vi "log analysis_gps.vi"() -> ()   [LabVIEW 2019] (continued)
02000000,471d,15824;INS_ALIGNMENT_COMPLETE,INS_RTKFIXED,37.37068318728,126.72136703307,8.7806,22.3000,0.4101,0.2924,-0.0105,-0.304454074,-0.851881109,32.302829580,0.4173,0.2841,0.5455,0.1136,0.0938,0.0834,0.2704,0.2490,5.0951,0f000001,0*5034c2f1\n\tsystem status\tnormal 2 28.200000 0 0\trobot status\t47.117309\t61.373325\t8.780600\t-0.304454\t-0.851881\t55.895889\t0.504000\t-0.016000\n\t\n15:08:15.2\tlog_raw\tgps_raw\t\tsystem status\tnormal 2 28.200000 0 0\trobot status\t47.257142\t61.573715\t8.772200\t-0.417275\t-0.794450\t55.326847\t0.500000\t-0.019000\n\t\n15:08:15.7\tlog_raw\tgps_raw\t\tsystem status\tnormal 2 28.200000 0 0\trobot status\t47.399461\t61.774255\t8.766600\t-0.526161\t-1.084867\t54.437000\t0.504000\t-0.024000\n\t\n15:08:16.2\tlog_raw\tgps_raw\t#INSPVAXA,USB3,0,45.5,FINESTEERING,2107,281314.250,02000000,471d,15824;INS_ALIGNMENT_COMPLETE,INS_RTKFIXED,37.37068860278,126.72137185474,8.7599,22.3000,0.3783,0.2883,-0.0099,-0.473451897,-1.199118445,33.419872159,0.4114,0.2852,0.5433,0.1126,0.0924,0.0813,0.2701,0.2485,5.0982,0f000001,0*254465a8\n\tsystem status\tnormal 2 28.200000 0 0\trobot status\t47.544405\t61.974360\t8.759900\t-0.473452\t-1.199118\t53.699936\t0.553000\t0.088000\n\t\n15:08:16.7\tlog_raw\tgps_raw\t#INSPVAXA,USB3,0,45.5,FINESTEERING,2107,281314.750,02000000,471d,15824;INS_ALIGNMENT_COMPLETE,INS_RTKFIXED,37.37069038063,126.72137348955,8.7529,22.3000,0.4019,0.3010,-0.0013,-0.576554942,-1.350073245,33.962253064,0.4114,0.2852,0.5433,0.1126,0.0924,0.0813,0.2701,0.2485,5.0982,0f000001,0*70de1d9e\n\tsystem status\tnormal 2 28.200000 0 0\trobot status\t47.689214\t62.171673\t8.752900\t-0.576555\t-1.350073\t53.539288\t0.494000\t-0.014000\n\t\n15:08:17.2\tlog_raw\tgps_raw\t\tsystem status\tnormal 2 28.200000 0 0\trobot status\t47.833567\t62.364346\t8.744900\t-0.295645\t-1.375257\t53.025951\t0.518000\t-0.006000\n\t\n15:08:17.7\tlog_raw\tgps_raw\t\tsystem status\tnormal 2 28.200000 0 0\trobot status\t47.974700\t62.554374\t8.738100\t-0.566007\t-1.595691\t51.924320\t0.511000\t0.009000\n\t\n15:08:18.2\tlog_raw\tgps_raw\t#INSPVAXA,USB3,0,50.0,FINESTEERING,2107,281316.250,02000000,471d,15824;INS_ALIGNMENT_COMPLETE,INS_RTKFIXED,37.37069553748,126.72137835296,8.7291,22.3000,0.3690,0.3016,-0.0165,-0.475362397,-1.709507066,35.267633649,0.4099,0.2844,0.5412,0.1123,0.0915,0.0796,0.2698,0.2480,5.0999,0f000001,0*7a9fb179\n\tsystem status\tnormal 2 28.200000 0 0\trobot status\t48.120006\t62.744002\t8.729100\t-0.475362\t-1.709507\t52.502842\t0.422000\t-0.071000\n\t\n15:08:18.7\tlog_raw\tgps_raw\t\tsystem status\tnormal 2 28.200000 0 0\trobot status\t48.271629\t62.938231\t8.721200\t-0.350668\t-1.662772\t52.101021\t0.431000\t-0.101000\n\t\n15:08:19.2\tlog_raw\tgps_raw\t#INSPVAXA,USB3,0,50.5,FINESTEERING,2107,281317.250,02000000,471d,15824;INS_ALIGNMENT_COMPLETE,INS_RTKFIXED,37.37069888473,126.72138166049,8.7140,22.3000,0.4002,0.3322,-0.0336,-0.163313359,-1.347458535,36.032748786,0.4094,0.2836,0.5396,0.1129,0.0921,0.0802,0.2696,0.2478,5.0996,0f000001,0*7e476d51\n\tsystem status\tnormal 2 28.200000 0 0\trobot status\t48.412982\t63.115493\t8.714000\t-0.163313\t-1.347459\t51.751701\t0.514000\t-0.007000\n\t\n15:08:19.7\tlog_raw\tgps_raw\t\tsystem status\tnormal 2 28.200000 0 0\trobot status\t48.561151\t63.300949\t8.706600\t-0.217369\t-1.146601\t51.645607\t0.473000\t-0.029000\n\t\n15:08:20.2\tlog_raw\tgps_raw\t#INSPVAXA,USB3,0,50.0,FINESTEERING,2107,281318.250,02000000,471d,15824;INS_ALIGNMENT_COMPLETE,INS_RTKFIXED,37.37070219067,126.72138499710,8.7014,22.3000,0.3959,0.3213,-0.0090,-0.394966992,-1.322496913,36.727773169,0.4088,0.2828,0.5369,0.1123,0.0917,0.0794,0.2695,0.2477,5.0989,0f000001,0*0ac65207\n\tsystem status\tnormal 2 28.200000 0 0\trobot status\t48.708533\t63.482400\t8.701400\t-0.394967\t-1.322497\t51.157326\t0.491000\t-0.005000\n\t\n15:08:20.7\tlog_raw\tgps_raw\t\tsystem status\tnormal 2 28.300000 0 0\trobot status\t48.862404\t63.669120\t8.695100\t-0.380069\t-1.561037\t50.880112\t0.497000\t0.006000\n\t\n15:08:21.2\tlog_raw\tgps_raw\t\tsystem status\tnormal 2 28.200000 0 0\trobot status\t49.009867\t63.846230\t8.690900\t-0.406987\t-1.733069\t50.231125\t0.491000\t0.004000\n\t\n15:08:21.7\tlog_raw\tgps_raw\t#INSPVAXA,USB3,0,48.5,FINESTEERING,2107,281319.750,02000000,471d,15824;INS_ALIGNMENT_COMPLETE,INS_RTKFIXED,37.37070705981,126.72139005862,8.6887,22.3000,0.3656,0.3184,-0.0246,-0.462020881,-1.503034844,37.411185291,0.4083,0.2820,0.5343,0.1120,0.0915,0.0787,0.2694,0.2475,5.0983,0f000001,0*abb76b38\n\tsystem status\tnormal 2 28.300000 0 0\trobot status\t49.156875\t64.022797\t8.688700\t-0.462021\t-1.503035\t50.616264\t0.494000\t0.013000\n\t\n15:08:22.2\tlog_raw\tgps_raw\t\tsystem status\tnormal 2 28.200000 0 0\trobot status\t49.308245\t64.205716\t8.683800\t-0.851405\t-1.203471\t49.388012\t0.496000\t0.022000\n\t\n15:08:22.7\tlog_raw\tgps_raw\t#INSPVAXA,USB3,0,48.5,FINESTEERING,2107,281320.750,02000000,471d,15824;INS_ALIGNMENT_COMPLETE,INS_RTKFIXED,37.37071031528,126.72139346401,8.6801,22.3000,0.3719,0.3343,-0.0256,-0.836621928,-1.161971448,37.866051675,0.4083,0.2824,0.5333,0.1117,0.0916,0.0783,0.2693,0.2474,5.0979,0f000001,0*4c0e47a3\n\tsystem status\tnormal 2 28.200000 0 0\trobot status\t49.458518\t64.384102\t8.680100\t-0.836622\t-1.161971\t50.094471\t0.500000\t-0.004000\n\t\n15:08:23.2\tlog_raw\tgps_raw\t\tsystem status\tnormal 2 28.200000 0 0\trobot status\t49.615893\t64.568116\t8.675800\t-0.658277\t-1.318533\t49.371201\t0.479000\t0.023000\n\t\n15:08:23.7\tlog_raw\tgps_raw\t\tsystem status\tnormal 2 28.200000 0 0\trobot status\t49.766057\t64.744809\t8.671200\t-0.776362\t-1.012949\t49.264000\t0.614000\t-0.157000\n\t\n15:08:24.2\tlog_raw\tgps_raw\t#INSPVAXA,USB3,0,47.0,FINESTEERING,2107,281322.250,02000000,471d,15824;INS_ALIGNMENT_COMPLETE,INS_RTKFIXED,37.37071517986,126.72139865405,8.6652,22.3000,0.3760,0.3375,-0.0171,-0.655763747,-1.033016654,37.379702834,0.4086,0.2835,0.5329,0.1123,0.0925,0.0785,0.2691,0.2470,5.0988,0f000001,0*f362831b\n\tsystem status\tnormal 2 28.200000 0 0\trobot status\t49.918244\t64.923993\t8.665200\t-0.655764\t-1.033017\t50.454414\t0.648000\t-0.215000\n\t\n15:08:24.7\tlog_raw\tgps_raw\t\tsystem status\tnormal 2 28.100000 0 0\trobot status\t50.066784\t65.103608\t8.660600\t-0.577701\t-1.081778\t51.485588\t0.625000\t-0.143000\n\t\n15:08:25.2\tlog_raw\tgps_raw\t\tsystem status\tnormal 2 28.100000 0 0\trobot status\t50.213324\t65.283613\t8.657100\t-0.452182\t-1.210138\t50.849743\t0.479000\t0.036000\n\t\n15:08:25.7\tlog_raw\tgps_raw\t#INSPVAXA,USB3,0,48.5,FINESTEERING,2107,281323.750,02000000,471d,15824;INS_ALIGNMENT_COMPLETE,INS_RTKFIXED,37.37072004459,126.72140359087,8.6528,22.3000,0.3627,0.2855,-0.0006,-0.403703824,-0.919601594,35.267300347,0.4085,0.2834,0.5316,0.1119,0.0920,0.0781,0.2688,0.2467,5.1000,0f000001,0*ec9c6181\n\tsystem status\tnormal 2 28.000000 0 0\trobot status\t50.355539\t65.463900\t8.652800\t-0.403704\t-0.919602\t51.615303\t0.379000\t0.207000\n\t\n15:08:26.2\tlog_raw\tgps_raw\t\tsystem status\tnormal 2 28.000000 0 0\trobot status\t50.496518\t65.649351\t8.648100\t-0.324737\t-0.975914\t53.271236\t0.348000\t0.245000\n\t\n15:08:26.7\tlog_raw\tgps_raw\t\tsystem status\tnormal 2 28.000000 0 0\trobot status\t50.634795\t65.837106\t8.645900\t-0.407789\t-1.128311\t53.314163\t0.459000\t0.079000\n\t\n15:08:27.2\tlog_raw\tgps_raw\t\tsystem status\tnormal 2 28.000000 0 0\trobot status\t50.769686\t66.027404\t8.642100\t-0.386832\t-1.074417\t55.010967\t0.361000\t0.214000\n\t\n15:08:27.7\tlog_raw\tgps_raw\t\tsystem status\tnormal 2 28.100000 0 0\trobot status\t50.902476\t66.219164\t8.636200\t-0.484459\t-1.076658\t55.567532\t0.427000\t0.099000\n\t\n15:08:28.2\tlog_raw\tgps_raw\t\tsystem status\tnormal 2 28.100000 0 0\trobot status\t51.036907\t66.415748\t8.630500\t-0.737464\t-1.315179\t55.762470\t0.474000\t0.058000\n\t\n15:08:28.7\tlog_raw\tgps_raw\t\tsystem status\tnormal 2 28.200000 0 0\trobot status\t51.171287\t66.612533\t8.623000\t-0.803976\t-1.518602\t55.944408\t0.455000\t0.055000\n\t\n15:08:29.2\tlog_raw\tgps_raw\t\tsystem status\tnormal 2 28.200000 0 0\trobot status\t51.302965\t66.808482\t8.615400\t-0.975887\t-1.577601\t55.492439\t0.415000\t0.109000\n\t\n15:08:29.7\tlog_raw\tgps_raw\t\tsystem status\tnormal 2 28.200000 0 0\trobot status\t51.436650\t67.003287\t8.608000\t-0.765257\t-1.468233\t55.661835\t0.471000\t0.022000\n\t\n15:08:30.2\tlog_raw\tgps_raw\t\tsystem status\tnormal 2 28.200000 0 0\trobot status\t51.569393\t67.199223\t8.602100\t-0.821984\t-1.470105\t56.289379\t0.476000\t-0.001000\n\t\n15:08:30.7\tlog_raw\tgps_raw\t\tsystem status\tnormal 2 28.200000 0 0\trobot status\t51.700644\t67.394092\t8.597100\t-0.936360\t-1.244626\t55.226109\t0.498000\t-0.010000\n\t\n15:08:31.2\tlog_raw\tgps_raw\t\tsystem status\tnormal 2 28.300000 0 0\trobot status\t51.836294\t67.592176\t8.591300\t-0.898016\t-1.271847\t55.102779\t0.483000\t-0.006000\n\t\n15:08:31.7\tlog_raw\tgps_raw\t\tsystem status\tnormal 2 28.200000 0 0\trobot status\t51.967517\t67.783831\t8.588300\t-0.834392\t-0.958625\t54.536842\t0.504000\t-0.006000\n\t\n15:08:32.2\tlog_raw\tgps_raw\t\tsystem status\tnormal 2 28.200000 0 0\trobot status\t52.104125\t67.983036\t8.585900\t-0.941680\t-1.166171\t54.890419\t0.489000\t-0.010000\n\t\n15:08:32.7\tlog_raw\tgps_raw\t\tsystem status\tnormal 2 28.200000 0 0\trobot status\t52.240414\t68.176706\t8.583300\t-0.898010\t-1.096168\t54.277641\t0.491000\t-0.017000\n\t\n15:08:33.2\tlog_raw\tgps_raw\t\tsystem status\tnormal 2 28.300000 0 0\trobot status\t52.379951\t68.372586\t8.581600\t-0.920489\t-1.314120\t54.206795\t0.495000\t-0.012000\n\t\n15:08:33.7\tlog_raw\tgps_raw\t\tsystem status\tnormal 2 28.200000 0 0\trobot status\t52.518260\t68.563321\t8.581200\t-1.159582\t-1.327353\t53.447784\t0.495000\t-0.017000\n\t\n15:08:34.2\tlog_raw\tgps_raw\t\tsystem status\tnormal 2 28.200000 0 0\trobot status\t52.661378\t68.752298\t8.580000\t-0.778607\t-1.287467\t53.848000\t0.495000\t-0.014000\n\t\n15:08:34.7\tlog_raw\tgps_raw\t\tsystem status\tnormal 2 28.200000 0 0\trobot status\t52.805205\t68.944887\t8.580000\t-0.943400\t-1.346339\t53.921986\t0.498000\t-0.014000\n\t\n15:08:35.2\tlog_raw\tgps_raw\t\tsystem status\tnormal 2 28.200000 0 0\trobot status\t52.948167\t69.137646\t8.579300\t-1.249705\t-1.354460\t53.620373\t0.494000\t-0.011000\n\t\n15:08:35.7\tlog_raw\tgps_raw\t\tsystem status\tnormal 2 28.200000 0 0\trobot status\t53.093231\t69.325947\t8.577100\t-1.029665\t-1.400629\t53.075745\t0.493000\t-0.012000\n\t\n15:08:36.2\tlog_raw\tgps_raw\t\tsystem status\tnormal 2 28.200000 0 0\trobot status\t53.237611\t69.513322\t8.576300\t-1.095579\t-1.217180\t52.815838\t0.490000\t-0.010000\n\t\n15:08:36.7\tlog_raw\tgps_raw\t\tsystem status\tnormal 2 28.200000 0 0\trobot status\t53.374531\t69.690053\t8.574000\t-1.352564\t-1.273880\t52.251175\t0.489000\t-0.006000\n\t\n15:08:37.2\tlog_raw\tgps_raw\t\tsystem status\tnormal 2 28.200000 0 0\trobot status\t53.525013\t69.879543\t8.571400\t-1.198409\t-1.204984\t51.399723\t0.497000\t-0.007000\n\t\n15:08:37.7\tlog_raw\tgps_raw\t\tsystem status\tnormal 2 28.200000 0 0\trobot status\t53.672559\t70.066195\t8.571500\t-1.318278\t-1.191439\t51.633030\t0.495000\t-0.004000\n\t\n15:08:38.2\tlog_raw\tgps_raw\t\tsystem status\tnormal 2 28.200000 0 0\trobot status\t53.813273\t70.242404\t8.572800\t-1.217463\t-1.069542\t50.886799\t0.491000\t0.004000\n\t\n15:08:38.7\tlog_raw\tgps_raw\t\tsystem status\tnormal 2 28.200000 0 0\trobot status\t53.957941\t70.426468\t8.575400\t-1.345030\t-1.058966\t51.660259\t0.489000\t0.001000\n\t\n15:08:39.2\tlog_raw\tgps_raw\t\tsystem status\tnormal 2 28.200000 0 0\trobot status\t54.110250\t70.616146\t8.576200\t-1.173305\t-1.126164\t52.342754\t0.504000\t0.002000\n\t\n15:08:39.7\tlog_raw\tgps_raw\t\tsystem status\tnormal 2 28.300000 0 0\trobot status\t54.256373\t70.797735\t8.577200\t-1.146366\t-0.932676\t51.256153\t0.499000\t0.004000\n\t\n15:08:40.2\tlog_raw\tgps_raw\t\tsystem status\tnormal 2 28.300000 0 0\trobot status\t54.407061\t70.984041\t8.578500\t-1.119779\t-1.061750\t53.940381\t0.510000\t-0.028000\n\t\n15:08:40.7\tlog_raw\tgps_raw\t\tsystem status\tnormal 2 28.200000 0 0\trobot status\t54.552738\t71.163348\t8.580300\t-1.072429\t-0.941882\t53.968372\t0.581000\t-0.117000\n\t\n15:08:41.2\tlog_raw\tgps_raw\t\tsystem status\tnormal 2 28.200000 0 0\trobot status\t54.700844\t71.350140\t8.581300\t-1.285029\t-0.941899\t54.047929\t0.602000\t-0.155000\n\t\n15:08:41.7\tlog_raw\tgps_raw\t\tsystem status\tnormal 2 28.200000 0 0\trobot status\t54.848417\t71.531667\t8.578000\t-1.210063\t-1.266019\t54.068840\t0.424000\t0.093000\n\t\n15:08:42.2\tlog_raw\tgps_raw\t\tsystem status\tnormal 2 28.200000 0 0\trobot status\t54.995909\t71.713856\t8.576000\t-1.122447\t-1.286200\t54.021425\t0.476000\t0.022000\n\t\n15:08:42.7\tlog_raw\tgps_raw\t\tsystem status\tnormal 2 28.200000 0 0\trobot status\t55.144573\t71.896954\t8.573500\t-0.954987\t-1.362437\t53.900030\t0.598000\t-0.132000\n\t\n15:08:43.3\tlog_raw\tgps_raw\t\tsystem status\tnormal 2 28.200000 0 0\trobot status\t55.290187\t72.076795\t8.572100\t-1.055723\t-1.303482\t53.917207\t0.444000\t0.068000\n\t\n15:08:43.8\tlog_raw\tgps_raw\t\tsystem status\tnormal 2 28.200000 0 0\trobot status\t55.439204\t72.259495\t8.571000\t-0.870480\t-1.490246\t53.889479\t0.467000\t0.026000\n\t\n15:08:44.3\tlog_raw\tgps_raw\t\tsystem status\tnormal 2 28.200000 0 0\trobot status\t55.583806\t72.438090\t8.570200\t-0.666404\t-1.298585\t53.950840\t0.588000\t-0.136000\n\t\n15:08:44.8\tlog_raw\tgps_raw\t\tsystem status\tnormal 2 28.200000 0 0\trobot status\t55.730372\t72.621257\t8.568500\t-0.702954\t-1.613137\t53.999544\t0.442000\t0.075000\n\t\n15:08:45.3\tlog_raw\tgps_raw\t\tsystem status\tnormal 2 28.200000 0 0\trobot status\t55.874225\t72.800761\t8.566900\t-0.755525\t-1.283546\t54.070638\t0.491000\t0.018000\n\t\n15:08:45.8\tlog_raw\tgps_raw\t\tsystem status\tnormal 2 28.200000 0 0\trobot status\t56.019116\t72.981255\t8.565000\t-0.800621\t-1.157915\t54.152009\t0.440000\t0.102000\n\t\n15:08:46.3\tlog_raw\tgps_raw\t\tsystem status\tnormal 2 28.200000 0 0\trobot status\t56.166448\t73.162692\t8.559900\t-0.704198\t-1.359800\t54.254209\t0.412000\t0.101000\n\t\n15:08:46.8\tlog_raw\tgps_raw\t\tsystem status\tnormal 2 28.200000 0 0\trobot status\t56.313046\t73.346457\t8.557700\t-0.959400\t-1.574238\t54.350406\t0.426000\t0.100000\n\t\n15:08:47.3\tlog_raw\tgps_raw\t\tsystem status\tnormal 2 28.200000 0 0\trobot status\t56.459141\t73.526626\t8.553900\t-0.675451\t-1.390689\t54.557566\t0.442000\t0.110000\n\t\n15:08:47.8\tlog_raw\tgps_raw\t\tsystem status\tnormal 2 28.200000 0 0\trobot status\t56.602807\t73.709315\t8.546800\t-0.785551\t-1.154932\t54.817335\t0.435000\t0.106000\n\t\n15:08:48.3\tlog_raw\tgps_raw\t\tsystem status\tnormal 2 28.200000 0 0\trobot status\t56.744703\t73.891677\t8.542100\t-0.819239\t-0.732265\t54.973358\t0.464000\t0.037000\n\t\n15:08:48.8\tlog_raw\tgps_raw\t\tsystem status\tnormal 2 28.200000 0 0\trobot status\t56.888549\t74.075432\t8.539300\t-0.665369\t-0.472677\t55.243402\t0.518000\t-0.059000\n\t\n15:08:49.3\tlog_raw\tgps_raw\t\tsystem status\tnormal 2 28.200000 0 0\trobot status\t57.031425\t74.265801\t8.535400\t-1.098864\t-0.638708\t55.361541\t0.494000\t0.003000\n\t\n15:08:49.8\tlog_raw\tgps_raw\t\tsystem status\tnormal 2 28.200000 0 0\trobot status\t57.176752\t74.455508\t8.530100\t-0.988437\t-0.701874\t55.591434\t0.446000\t0.053000\n\t\n15:08:50.3\tlog_raw\tgps_raw\t\tsystem status\tnormal 2 28.200000 0 0\trobot status\t57.319183\t74.646454\t8.524900\t-1.121493\t-0.989373\t55.778627\t0.489000\t0.014000\n\t\n15:08:50.8\tlog_raw\tgps_raw\t\tsystem status\tnormal 2 28.200000 0 0\trobot status\t57.461603\t74.839493\t8.519000\t-1.123970\t-0.950468\t55.854304\t0.398000\t0.137000\n\t\n15:08:51.3\tlog_raw\tgps_raw\t\tsystem status\tnormal 2 28.200000 0 0\trobot status\t57.601461\t75.031968\t8.514100\t-1.256286\t-1.067505\t55.924902\t0.606000\t-0.155000\n\t\n15:08:51.8\tlog_raw\tgps_raw\t\tsystem status\tnormal 2 28.200000 0 0\trobot status\t57.745208\t75.224870\t8.511200\t-1.174015\t-1.121104\t55.982848\t0.611000\t-0.175000\n\t\n15:08:52.3\tlog_raw\tgps_raw\t#INSPVAXA,USB3,0,48.0,FINESTEERING,2107,281350.300,02000000,471d,15824;INS_ALIGNMENT_COMPLETE,INS_RTKFIXED,37.37080986573,126.72148875740,8.5075,22.3000,0.3628,0.2976,-0.0057,-1.206867274,-0.983762536,33.908435264,0.4194,0.3028,0.5790,0.1129,0.0949,0.0832,0.2672,0.2431,5.1219,0f000001,0*073b2b30\n\tsystem status\tnormal 2 28.200000 0 0\trobot status\t57.899451\t75.432615\t8.507500\t-1.206867\t-0.983763\t56.091565\t0.472000\t0.044000\n\t\n15:08:52.8\tlog_raw\tgps_raw\t\tsystem status\tnormal 2 28.200000 0 0\trobot status\t58.029433\t75.607614\t8.505000\t-1.226590\t-0.870732\t56.099036\t0.428000\t0.083000\n\t\n15:08:53.3\tlog_raw\tgps_raw\t\tsystem status\tnormal 2 28.200000 0 0\trobot status\t58.172374\t75.798762\t8.502200\t-1.085314\t-0.848548\t56.025604\t0.498000\t-0.012000\n\t\n15:08:53.8\tlog_raw\tgps_raw\t#INSPVAXA,USB3,0,48.0,FINESTEERING,2107,281351.800,02000000,471d,15824;INS_ALIGNMENT_COMPLETE,INS_RTKFIXED,37.37081508694,126.72149360654,8.4972,22.3000,0.3531,0.2937,-0.0017,-1.250896951,-0.823004101,34.091002532,0.4207,0.3049,0.5833,0.1126,0.0947,0.0826,0.2672,0.2430,5.1224,0f000001,0*3c5ad9c3\n\tsystem status\tnormal 2 28.200000 0 0\trobot status\t58.328980\t76.012086\t8.497200\t-1.250897\t-0.823004\t55.908997\t0.506000\t-0.023000\n\t\n15:08:54.3\tlog_raw\tgps_raw\t\tsystem status\tnormal 2 28.200000 0 0\trobot status\t58.456743\t76.183693\t8.494600\t-1.140373\t-0.821052\t55.816580\t0.484000\t0.008000\n\t\n15:08:54.8\tlog_raw\tgps_raw\t\tsystem status\tnormal 2 28.200000 0 0\trobot status\t58.600409\t76.376434\t8.488900\t-0.942472\t-0.841260\t55.732045\t0.512000\t-0.021000\n\t\n15:08:55.3\tlog_raw\tgps_raw\t\tsystem status\tnormal 2 28.200000 0 0\trobot status\t58.740471\t76.564815\t8.485800\t-1.089114\t-0.807718\t55.658014\t0.491000\t0.002000\n\t\n15:08:55.8\tlog_raw\tgps_raw\t\tsystem status\tnormal 2 28.200000 0 0\trobot status\t58.889135\t76.760157\t8.483300\t-0.717967\t-1.020213\t55.563477\t0.495000\t-0.005000\n\t\n15:08:56.3\tlog_raw\tgps_raw\t\tsystem status\tnormal 2 28.200000 0 0\trobot status\t59.031386\t76.953603\t8.478900\t-1.103324\t-1.081036\t55.464401\t0.495000\t0.000000\n\t\n15:08:56.8\tlog_raw\tgps_raw\t\tsystem status\tnormal 2 28.200000 0 0\trobot status\t59.176177\t77.146597\t8.475300\t-1.136420\t-1.065385\t55.315970\t0.498000\t-0.014000\n\t\n15:08:57.3\tlog_raw\tgps_raw\t\tsystem status\tnormal 2 28.200000 0 0\trobot status\t59.323529\t77.338500\t8.470600\t-0.820529\t-1.007914\t55.132802\t0.504000\t-0.013000\n\t\n15:08:57.8\tlog_raw\tgps_raw\t#INSPVAXA,USB3,0,49.0,FINESTEERING,2107,281355.800,02000000,471d,15824;INS_ALIGNMENT_COMPLETE,INS_RTKFIXED,37.37082893700,126.72150664306,8.4666,22.3000,0.3730,0.3109,-0.0009,-1.161970784,-1.138060141,34.996264200,0.4190,0.3015,0.5793,0.1125,0.0944,0.0820,0.2670,0.2425,5.1250,0f000001,0*10c36a68\n\tsystem status\tnormal 2 28.200000 0 0\trobot status\t59.483733\t77.549221\t8.466600\t-1.161971\t-1.138060\t55.003736\t0.499000\t-0.010000\n\t\n15:08:58.3\tlog_raw\tgps_raw\t#INSPVAXA,USB3,0,48.0,FINESTEERING,2107,281356.300,02000000,471d,15824;INS_ALIGNMENT_COMPLETE,INS_RTKFIXED,37.37083063572,126.72150829045,8.4620,22.3000,0.3521,0.3106,-0.0162,-1.118678244,-0.900069608,35.100092302,0.4187,0.3015,0.5781,0.1134,0.0955,0.0834,0.2669,0.2424,5.1261,0f000001,0*ecce3653\n\tsystem status\tnormal 2 28.200000 0 0\trobot status\t59.629656\t77.737752\t8.462000\t-1.118678\t-0.900070\t54.899908\t0.502000\t0.005000\n\t\n15:08:58.8\tlog_raw\tgps_raw\t#INSPVAXA,USB3,0,48.0,FINESTEERING,2107,281356.800,02000000,471d,15824;INS_ALIGNMENT_COMPLETE,INS_RTKFIXED,37.37083231067,126.72150995992,8.4554,22.3000,0.3495,0.3060,0.0042,-0.932722694,-0.812097133,35.195809963,0.4187,0.3015,0.5781,0.1134,0.0955,0.0834,0.2669,0.2424,5.1261,0f000001,0*f7e2c3ce\n\tsystem status\tnormal 2 28.200000 0 0\trobot status\t59.777535\t77.923645\t8.455400\t-0.932723\t-0.812097\t54.804190\t0.499000\t-0.003000\n\t\n15:08:59.3\tlog_raw\tgps_raw\t\tsystem status\tnormal 2 28.200000 0 0\trobot status\t59.910515\t78.091903\t8.450900\t-0.858521\t-0.877630\t54.774911\t0.495000\t-0.004000\n\t\n15:08:59.8\tlog_raw\tgps_raw\t\tsystem status\tnormal 2 28.200000 0 0\trobot status\t60.056948\t78.279781\t8.445500\t-1.000569\t-0.920241\t54.626841\t0.507000\t-0.016000\n\t\n15:09:00.3\tlog_raw\tgps_raw\t#INSPVAXA,USB3,0,47.5,FINESTEERING,2107,281358.300,02000000,471d,15824;INS_ALIGNMENT_COMPLETE,INS_RTKFIXED,37.37083738053,126.72151493365,8.4383,22.3000,0.3581,0.3251,0.0034,-0.998984174,-0.973141435,35.285574115,0.4158,0.2963,0.5677,0.1128,0.0943,0.0826,0.2668,0.2421,5.1287,0f000001,0*5ae881cd\n\tsystem status\tnormal 2 28.200000 0 0\trobot status\t60.218100\t78.486318\t8.438300\t-0.998984\t-0.973141\t54.714426\t0.575000\t-0.122000\n\t\n15:09:00.8\tlog_raw\tgps_raw\t#INSPVAXA,USB3,0,47.5,FINESTEERING,2107,281358.800,02000000,471d,15824;INS_ALIGNMENT_COMPLETE,INS_RTKFIXED,37.37083909479,126.72151662067,8.4311,22.3000,0.3558,0.3072,-0.0005,-0.868229023,-1.222380492,35.266513132,0.4158,0.2963,0.5677,0.1128,0.0943,0.0826,0.2668,0.2421,5.1287,0f000001,0*f5ce0274\n\tsystem status\tnormal 2 28.200000 0 0\trobot status\t60.367534\t78.676573\t8.431100\t-0.868229\t-1.222380\t54.733487\t0.418000\t0.122000\n\t\n15:09:01.3\tlog_raw\tgps_raw\t\tsystem status\tnormal 2 28.200000 0 0\trobot status\t60.499909\t78.845706\t8.425500\t-0.880542\t-1.139747\t54.853674\t0.453000\t0.077000\n\t\n15:09:01.8\tlog_raw\tgps_raw\t\tsystem status\tnormal 2 28.200000 0 0\trobot status\t60.645231\t79.032334\t8.421200\t-0.872036\t-1.156870\t54.900207\t0.475000\t0.036000\n\t\n15:09:02.3\tlog_raw\tgps_raw\t#DUALANTENNAHEADINGA,USB3,0,49.0,FINESTEERING,2107,281360.300,02000000,d426,15824;SOL_COMPUTED,NARROW_FLOAT,-1.000000000,43.377029419,-28.936859131,0.0,317.200378418,180.000000000,\"631T\",19,9,9,8,04,00,20,03*d052c393\n\tsystem status\tnormal 2 28.200000 0 0\trobot status\t60.808916\t79.242566\t8.414700\t-0.856033\t-1.140138\t55.073601\t0.605000\t-0.162000\n\t\n15:09:02.8\tlog_raw\tgps_raw\t#DUALANTENNAHEADINGA,USB3,0,49.0,FINESTEERING,2107,281360.800,02000000,d426,15824;SOL_COMPUTED,NARROW_FLOAT,-1.000000000,41.997791290,-30.735473633,0.0,321.670349121,180.000000000,\"631T\",18,9,9,8,04,00,20,03*cef783d0\n\tsystem status\tnormal 2 28.200000 0 0\trobot status\t60.953139\t79.430817\t8.410100\t-0.877008\t-1.314238\t55.106052\t0.601000\t-0.157000\n\t\n15:09:03.3\tlog_raw\tgps_raw\t#DUALANTENNAHEADINGA,USB3,0,46.5,FINESTEERING,2107,281361.300,02000000,d426,15824;SOL_COMPUTED,NARROW_FLOAT,-1.000000000,39.328605652,-30.210357666,0.0,354.292755127,180.000000000,\"631T\",19,9,9,8,04,00,20,03*65c8eaaf\n\tsystem status\tnormal 2 28.200000 0 0\trobot status\t61.099056\t79.619660\t8.404400\t-0.730402\t-1.313099\t55.284228\t0.431000\t0.103000\n\t\n15:09:03.8\tlog_raw\tgps_raw\t#INSPVAXA,USB3,0,46.5,FINESTEERING,2107,281361.800,02000000,471d,15824;INS_ALIGNMENT_COMPLETE,INS_RTKFIXED,37.37084928466,126.72152648987,8.4001,22.3000,0.3666,0.2894,0.0007,-0.918254878,-1.223429977,34.701580667,0.4179,0.3011,0.5737,0.1121,0.0941,0.0814,0.2668,0.2419,5.1323,0f000001,0*40ddb97a\n\tsystem status\tnormal 2 28.200000 0 0\trobot status\t61.241731\t79.807486\t8.400100\t-0.918255\t-1.223430\t55.298419\t0.576000\t-0.120000\n\t\n15:09:04.3\tlog_raw\tgps_raw\t#DUALANTENNAHEADINGA,USB3,0,48.0,FINESTEERING,2107,281362.300,02000000,d426,15824;SOL_COMPUTED,NARROW_FLOAT,-1.000000000,51.965854645,-24.394927979,0.0,236.640274048,180.000000000,\"631T\",19,9,9,8,04,00,20,03*62047533\n\tsystem status\tnormal 2 28.200000 0 0\trobot status\t61.388512\t80.001930\t8.394700\t-0.918081\t-1.262897\t55.420377\t0.460000\t0.037000\n\t\n15:09:04.8\tlog_raw\tgps_raw\t#DUALANTENNAHEADINGA,USB3,0,48.0,FINESTEERING,2107,281362.800,02000000,d426,15824;SOL_COMPUTED,NARROW_FLOAT,-1.000000000,51.700309753,-22.485168457,0.0,233.081008911,180.000000000,\"631T\",19,9,9,8,04,00,20,03*ce0df6af\n\tsystem status\tnormal 2 28.200000 0 0\trobot status\t61.530927\t80.190999\t8.388800\t-0.881646\t-1.493081\t55.555090\t0.488000\t0.017000\n\t\n15:09:05.3\tlog_raw\tgps_raw\t#DUALANTENNAHEADINGA,USB3,0,46.0,FINESTEERING,2107,281363.300,02000000,d426,15824;SOL_COMPUTED,NARROW_FLOAT,-1.000000000,37.930927277,-27.303833008,0.0,334.334472656,180.000000000,\"631T\",20,9,9,7,04,00,20,03*296cd207\n\tsystem status\tnormal 2 28.200000 0 0\trobot status\t61.674515\t80.381791\t8.384900\t-0.875859\t-1.426274\t55.582554\t0.589000\t-0.152000\n\t\n15:09:05.8\tlog_raw\tgps_raw\t#DUALANTENNAHEADINGA,USB3,0,46.0,FINESTEERING,2107,281363.800,02000000,d426,15824;SOL_COMPUTED,NARROW_FLOAT,-1.000000000,38.201625824,-27.727355957,0.0,332.017791748,180.000000000,\"631T\",23,9,9,8,04,00,20,03*f0493f23\n\tsystem status\tnormal 2 28.200000 0 0\trobot status\t61.819190\t80.574203\t8.379100\t-0.630472\t-1.495988\t55.589533\t0.427000\t0.087000\n\t\n15:09:06.3\tlog_raw\tgps_raw\t#DUALANTENNAHEADINGA,USB3,0,44.0,FINESTEERING,2107,281364.300,02000000,d426,15824;SOL_COMPUTED,NARROW_FLOAT,-1.000000000,49.235725403,-25.915039063,0.0,256.086944580,180.000000000,\"631T\",24,9,9,8,04,00,20,03*6ae9d837\n\tsystem status\tnormal 2 28.300000 0 0\trobot status\t61.961259\t80.766328\t8.373600\t-0.632140\t-1.345250\t55.599970\t0.433000\t0.102000\n\t\n15:09:06.8\tlog_raw\tgps_raw\t#INSPVAXA,USB3,0,44.0,FINESTEERING,2107,281364.800,02000000,471d,15824;INS_ALIGNMENT_COMPLETE,INS_RTKFIXED,37.37085965164,126.72153621397,8.3672,22.3000,0.3702,0.3004,-0.0120,-0.629392429,-1.475289805,34.330847261,0.4175,0.2991,0.5747,0.1118,0.0936,0.0803,0.2665,0.2416,5.1319,0f000001,0*907d57c4\n\tsystem status\tnormal 2 28.200000 0 0\trobot status\t62.103076\t80.958054\t8.367200\t-0.629392\t-1.475290\t55.669153\t0.414000\t0.118000\n\t\n15:09:07.3\tlog_raw\tgps_raw\t#DUALANTENNAHEADINGA,USB3,0,48.0,FINESTEERING,2107,281365.300,02000000,d426,15824;SOL_COMPUTED,NARROW_FLOAT,-1.000000000,46.742221832,-24.611022949,0.0,308.216918945,180.000000000,\"631T\",18,9,9,8,04,00,20,03*16f83fc7\n\tsystem status\tnormal 2 28.200000 0 0\trobot status\t62.245896\t81.147823\t8.360800\t-0.307441\t-1.510534\t55.703119\t0.440000\t0.084000\n\t\n15:09:07.8\tlog_raw\tgps_raw\t#DUALANTENNAHEADINGA,USB3,0,48.0,FINESTEERING,2107,281365.800,02000000,d426,15824;SOL_COMPUTED,NARROW_FLOAT,-1.000000000,45.876544952,-25.206176758,0.0,301.727966309,180.000000000,\"631T\",19,9,9,8,04,00,20,03*878e3cfa\n\tsystem status\tnormal 2 28.200000 0 0\trobot status\t62.386948\t81.338395\t8.355400\t-0.446797\t-1.535601\t55.711159\t0.572000\t-0.123000\n\t\n15:09:08.3\tlog_raw\tgps_raw\t#INSPVAXA,USB3,0,50.0,FINESTEERING,2107,281366.300,02000000,471d,15824;INS_ALIGNMENT_COMPLETE,INS_RTKFIXED,37.37086481879,126.72154103574,8.3492,22.3000,0.3841,0.2933,-0.0130,-0.540868347,-1.307063717,34.323850336,0.4168,0.2979,0.5715,0.1114,0.0932,0.0794,0.2664,0.2414,5.1301,0f000001,0*c00b2394\n\tsystem status\tnormal 2 28.200000 0 0\trobot status\t62.530181\t81.531525\t8.349200\t-0.540868\t-1.307064\t55.676150\t0.600000\t-0.149000\n\t\n15:09:08.8\tlog_raw\tgps_raw\t#INSPVAXA,USB3,0,50.0,FINESTEERING,2107,281366.800,02000000,471d,15824;INS_ALIGNMENT_COMPLETE,INS_RTKFIXED,37.37086653652,126.72154262606,8.3447,22.3000,0.3779,0.3041,-0.0177,-0.586317091,-1.274041965,34.268661727,0.4168,0.2979,0.5715,0.1114,0.0932,0.0794,0.2664,0.2414,5.1301,0f000001,0*197e2cdd\n\tsystem status\tnormal 2 28.200000 0 0\trobot status\t62.671049\t81.722166\t8.344700\t-0.586317\t-1.274042\t55.731338\t0.432000\t0.091000\n\t\n15:09:09.3\tlog_raw\tgps_raw\t#DUALANTENNAHEADINGA,USB3,0,48.0,FINESTEERING,2107,281367.300,02000000,d426,15824;SOL_COMPUTED,NARROW_FLOAT,-1.000000000,57.061241150,-31.246337891,0.0,140.264724731,180.000000000,\"631T\",19,11,11,8,04,00,30,03*83af5acf\n\tsystem status\tnormal 2 28.200000 0 0\trobot status\t62.811207\t81.912480\t8.341000\t-0.562255\t-1.090376\t55.713331\t0.465000\t0.033000\n\t\n15:09:09.8\tlog_raw\tgps_raw\t#DUALANTENNAHEADINGA,USB3,0,48.0,FINESTEERING,2107,281367.800,02000000,d426,15824;SOL_COMPUTED,NARROW_FLOAT,-1.000000000,57.968719482,-32.427215576,0.0,139.111709595,180.000000000,\"631T\",22,11,11,8,04,00,30,03*64b77029\n\tsystem status\tnormal 2 28.200000 0 0\trobot status\t62.951214\t82.103953\t8.339200\t-0.675245\t-0.949264\t55.659939\t0.590000\t-0.140000\n\t\n15:09:10.3\tlog_raw\tgps_raw\t#INSPVAXA,USB3,0,45.0,FINESTEERING,2107,281368.300,02000000,471d,15824;INS_ALIGNMENT_COMPLETE,INS_RTKFIXED,37.37087168794,126.72154735160,8.3372,22.3000,0.3761,0.3168,-0.0092,-0.837699273,-0.815511230,34.270342618,0.4149,0.2944,0.5637,0.1114,0.0930,0.0792,0.2662,0.2411,5.1296,0f000001,0*cf514333\n\tsystem status\tnormal 2 28.200000 0 0\trobot status\t63.089629\t82.293891\t8.337200\t-0.837699\t-0.815511\t55.729657\t0.439000\t0.082000\n\t\n15:09:10.8\tlog_raw\tgps_raw\t#INSPVAXA,USB3,0,45.0,FINESTEERING,2107,281368.800,02000000,471d,15824;INS_ALIGNMENT_COMPLETE,INS_RTKFIXED,37.37087344572,126.72154897754,8.3331,22.3000,0.3716,0.2920,0.0040,-0.667583562,-0.920128671,34.279798590,0.4149,0.2944,0.5637,0.1114,0.0930,0.0792,0.2662,0.2411,5.1296,0f000001,0*f456fa2a\n\tsystem status\tnormal 2 28.200000 0 0\trobot status\t63.233652\t82.488977\t8.333100\t-0.667584\t-0.920129\t55.720201\t0.429000\t0.085000\n\t\n15:09:11.3\tlog_raw\tgps_raw\t#DUALANTENNAHEADINGA,USB3,0,47.0,FINESTEERING,2107,281369.300,02000000,d426,15824;SOL_COMPUTED,NARROW_FLOAT,-1.000000000,48.869911194,-23.291656494,0.0,246.362884521,180.000000000,\"631T\",19,9,9,8,04,00,20,03*fdb2b4cf\n\tsystem status\tnormal 2 28.200000 0 0\trobot status\t63.372996\t82.679380\t8.329400\t-0.672586\t-0.863596\t55.701930\t0.572000\t-0.122000\n\t\n15:09:11.8\tlog_raw\tgps_raw\t#INSPVAXA,USB3,0,47.0,FINESTEERING,2107,281369.800,02000000,471d,15824;INS_ALIGNMENT_COMPLETE,INS_RTKFIXED,37.37087693639,126.72155218192,8.3258,22.3000,0.3824,0.3082,-0.0032,-0.585559020,-1.104223780,34.420056753,0.4144,0.2935,0.5605,0.1112,0.0927,0.0788,0.2662,0.2410,5.1304,0f000001,0*fed5d425\n\tsystem status\tnormal 2 28.200000 0 0\trobot status\t63.517491\t82.876385\t8.325800\t-0.585559\t-1.104224\t55.579943\t0.504000\t-0.006000\n\t\n15:09:12.3\tlog_raw\tgps_raw\t#DUALANTENNAHEADINGA,USB3,0,48.5,FINESTEERING,2107,281370.300,02000000,d426,15824;SOL_COMPUTED,NARROW_FLOAT,-1.000000000,56.995876312,-45.029174805,0.0,226.826354980,180.000000000,\"631T\",18,8,8,8,04,00,20,03*06abc766\n\tsystem status\tnormal 2 28.200000 0 0\trobot status\t63.657787\t83.063346\t8.322800\t-0.510550\t-1.263076\t55.509939\t0.495000\t-0.009000\n\t\n15:09:12.8\tlog_raw\tgps_raw\t#DUALANTENNAHEADINGA,USB3,0,48.5,FINESTEERING,2107,281370.800,02000000,d426,15824;SOL_COMPUTED,NARROW_FLOAT,-1.000000000,56.755435944,-45.314361572,0.0,225.346038818,180.000000000,\"631T\",19,8,8,8,04,00,20,03*c8312a5e\n\tsystem status\tnormal 2 28.200000 0 0\trobot status\t63.804879\t83.255330\t8.321200\t-0.435831\t-1.146017\t55.376461\t0.503000\t-0.025000\n\t\n15:09:13.3\tlog_raw\tgps_raw\t\tsystem status\tnormal 2 28.200000 0 0\trobot status\t63.946253\t83.441804\t8.317400\t-0.497326\t-1.069834\t55.299111\t0.494000\t0.001000\n\t\n15:09:13.8\tlog_raw\tgps_raw\t#DUALANTENNAHEADINGA,USB3,0,47.5,FINESTEERING,2107,281371.800,02000000,d426,15824;SOL_COMPUTED,NARROW_FLOAT,-1.000000000,65.830406189,-48.192810059,0.0,160.190460205,180.000000000,\"631T\",20,8,8,8,04,00,20,03*a1e2e423\n\tsystem status\tnormal 2 28.200000 0 0\trobot status\t64.090380\t83.628170\t8.314200\t-0.085380\t-1.102762\t55.241580\t0.492000\t0.002000\n\t\n15:09:14.3\tlog_raw\tgps_raw\t#DUALANTENNAHEADINGA,USB3,0,51.0,FINESTEERING,2107,281372.300,02000000,d426,15824;SOL_COMPUTED,NARROW_FLOAT,-1.000000000,46.303096771,-16.665802002,0.0,249.117385864,180.000000000,\"631T\",21,9,9,8,04,00,20,03*9ebf37bc\n\tsystem status\tnormal 2 28.200000 0 0\trobot status\t64.228704\t83.811888\t8.311300\t-0.407735\t-0.837486\t55.181323\t0.575000\t-0.118000\n\t\n15:09:14.8\tlog_raw\tgps_raw\t#DUALANTENNAHEADINGA,USB3,0,51.0,FINESTEERING,2107,281372.800,02000000,d426,15824;SOL_COMPUTED,NARROW_FLOAT,-1.000000000,47.137203217,-16.407073975,0.0,245.953109741,180.000000000,\"631T\",21,9,9,8,04,00,20,03*e468614e\n\tsystem status\tnormal 2 28.200000 0 0\trobot status\t64.370827\t84.002947\t8.306400\t-0.663117\t-0.964402\t55.186069\t0.439000\t0.070000\n\t\n15:09:15.3\tlog_raw\tgps_raw\t#DUALANTENNAHEADINGA,USB3,0,48.0,FINESTEERING,2107,281373.300,02000000,d426,15824;SOL_COMPUTED,NARROW_FLOAT,-1.000000000,40.694911957,-17.624786377,0.0,282.511657715,180.000000000,\"631T\",21,9,9,8,04,00,20,03*fc4a9f69\n\tsystem status\tnormal 2 28.200000 0 0\trobot status\t64.514373\t84.190714\t8.302000\t-0.474336\t-1.249125\t55.204782\t0.471000\t0.023000\n\t\n15:09:15.8\tlog_raw\tgps_raw\t#DUALANTENNAHEADINGA,USB3,0,48.0,FINESTEERING,2107,281373.800,02000000,d426,15824;SOL_COMPUTED,NARROW_FLOAT,-1.000000000,39.396804810,-18.797271729,0.0,283.153411865,180.000000000,\"631T\",22,9,9,8,04,00,20,03*8a178ec6\n\tsystem status\tnormal 2 28.200000 0 0\trobot status\t64.656120\t84.377141\t8.300100\t-0.646463\t-1.247567\t55.165851\t0.590000\t-0.130000\n\t\n15:09:16.3\tlog_raw\tgps_raw\t\tsystem status\tnormal 2 28.200000 0 0\trobot status\t64.798285\t84.562825\t8.297000\t-0.531319\t-1.269823\t55.188044\t0.577000\t-0.132000\n\t\n15:09:16.8\tlog_raw\tgps_raw\t#DUALANTENNAHEADINGA,USB3,0,45.0,FINESTEERING,2107,281374.800,02000000,d426,15824;SOL_COMPUTED,NARROW_FLOAT,-1.000000000,39.349189758,-20.650939941,0.0,277.168212891,180.000000000,\"631T\",22,9,9,8,04,00,20,03*f8ab3252\n\tsystem status\tnormal 2 28.200000 0 0\trobot status\t64.940908\t84.753570\t8.294900\t-0.658703\t-1.274906\t55.231582\t0.605000\t-0.165000\n\t\n15:09:17.3\tlog_raw\tgps_raw\t#DUALANTENNAHEADINGA,USB3,0,44.5,FINESTEERING,2107,281375.300,02000000,d426,15824;SOL_COMPUTED,NARROW_FLOAT,-1.000000000,34.529243469,-20.115325928,0.0,317.339965820,180.000000000,\"631T\",22,9,9,8,04,00,20,03*a594d36f\n\tsystem status\tnormal 2 28.200000 0 0\trobot status\t65.081470\t84.937748\t8.293300\t-0.695336\t-1.169688\t55.303485\t0.435000\t0.089000\n\t\n15:09:17.8\tlog_raw\tgps_raw\t#DUALANTENNAHEADINGA,USB3,0,44.5,FINESTEERING,2107,281375.800,02000000,d426,15824;SOL_COMPUTED,NARROW_FLOAT,-1.000000000,34.753417969,-19.800323486,0.0,315.846893311,180.000000000,\"631T\",22,9,9,8,04,00,20,03*6b0303b2\n\tsystem status\tnormal 2 28.200000 0 0\trobot status\t65.225290\t85.123740\t8.289600\t-0.507901\t-0.973672\t55.458271\t0.464000\t0.052000\n\t\n15:09:18.3\tlog_raw\tgps_raw\t#DUALANTENNAHEADINGA,USB3,0,46.0,FINESTEERING,2107,281376.300,02000000,d426,15824;SOL_COMPUTED,NARROW_FLOAT,-1.000000000,41.617706299,-20.286529541,0.0,249.996673584,180.000000000,\"631T\",22,9,9,8,04,00,20,03*8e0e78c9\n\tsystem status\tnormal 2 28.200000 0 0\trobot status\t65.368510\t85.309571\t8.285800\t-0.251511\t-1.084942\t55.598201\t0.596000\t-0.149000\n\t\n15:09:18.8\tlog_raw\tgps_raw\t\tsystem status\tnormal 2 28.200000 0 0\trobot status\t65.510469\t85.498896\t8.282600\t-0.383999\t-1.117773\t55.654076\t0.495000\t0.006000\n\t\n15:09:19.3\tlog_raw\tgps_raw\t#DUALANTENNAHEADINGA,USB3,0,45.0,FINESTEERING,2107,281377.300,02000000,d426,15824;SOL_COMPUTED,NARROW_FLOAT,-1.000000000,38.012714386,-20.573577881,0.0,307.964691162,180.000000000,\"631T\",20,9,9,8,04,00,20,03*3937b18a\n\tsystem status\tnormal 2 28.200000 0 0\trobot status\t65.653366\t85.687915\t8.278600\t-0.451237\t-1.194223\t55.758623\t0.419000\t0.116000\n\t\n15:09:19.8\tlog_raw\tgps_raw\t#DUALANTENNAHEADINGA,USB3,0,45.0,FINESTEERING,2107,281377.800,02000000,d426,15824;SOL_COMPUTED,NARROW_FLOAT,-1.000000000,38.498992920,-20.027069092,0.0,303.899200439,180.000000000,\"631T\",20,9,9,8,04,00,20,03*e32a34d5\n\tsystem status\tnormal 2 28.200000 0 0\trobot status\t65.795423\t85.874279\t8.275100\t-0.328526\t-0.992598\t55.985701\t0.470000\t0.034000\n\t\n15:09:20.3\tlog_raw\tgps_raw\t#DUALANTENNAHEADINGA,USB3,0,49.5,FINESTEERING,2107,281378.300,02000000,d426,15824;SOL_COMPUTED,NARROW_FLOAT,-1.000000000,27.239126205,-17.903564453,0.0,360.000000000,180.000000000,\"631T\",20,9,9,8,04,00,20,03*3fff5ac6\n\tsystem status\tnormal 2 28.200000 0 0\trobot status\t65.936214\t86.061320\t8.272100\t-0.436630\t-0.692866\t56.071896\t0.415000\t0.106000\n\t\n15:09:20.8\tlog_raw\tgps_raw\t\tsystem status\tnormal 2 28.200000 0 0\trobot status\t66.079189\t86.250636\t8.266000\t-0.558490\t-0.993340\t56.262711\t0.574000\t-0.119000\n\t\n15:09:21.3\tlog_raw\tgps_raw\t#DUALANTENNAHEADINGA,USB3,0,48.5,FINESTEERING,2107,281379.300,02000000,d426,15824;SOL_COMPUTED,NARROW_FLOAT,-1.000000000,30.153203964,-39.951202393,0.0,341.163116455,180.000000000,\"631T\",22,8,8,8,04,00,20,03*fe3aefcd\n\tsystem status\tnormal 2 28.200000 0 0\trobot status\t66.221378\t86.441558\t8.261700\t-0.739684\t-1.059339\t56.311479\t0.496000\t0.006000\n\t\n15:09:21.8\tlog_raw\tgps_raw\t\tsystem status\tnormal 2 28.200000 0 0\trobot status\t66.360800\t86.631908\t8.257800\t-1.037488\t-1.206723\t56.323102\t0.621000\t-0.169000\n\t\n15:09:22.3\tlog_raw\tgps_raw\t#DUALANTENNAHEADINGA,USB3,0,47.5,FINESTEERING,2107,281380.300,02000000,d426,15824;SOL_COMPUTED,NARROW_FLOAT,-1.000000000,31.592365265,-19.809661865,0.0,316.837921143,180.000000000,\"631T\",19,9,9,8,04,00,20,03*09fa2adc\n\tsystem status\tnormal 2 28.200000 0 0\trobot status\t66.502511\t86.820251\t8.253600\t-0.732331\t-1.246821\t56.348361\t0.565000\t-0.126000\n\t\n15:09:22.8\tlog_raw\tgps_raw\t\tsystem status\tnormal 2 28.200000 0 0\trobot status\t66.642790\t87.013104\t8.248800\t-1.028766\t-1.287518\t56.347518\t0.568000\t-0.126000\n\t\n15:09:23.3\tlog_raw\tgps_raw\t#DUALANTENNAHEADINGA,USB3,0,46.0,FINESTEERING,2107,281381.300,02000000,d426,15824;SOL_COMPUTED,NARROW_FLOAT,-1.000000000,31.278856277,-21.390625000,0.0,327.912139893,180.000000000,\"631T\",19,9,9,8,04,00,20,03*4fc11f4c\n\tsystem status\tnormal 2 28.200000 0 0\trobot status\t66.786498\t87.206784\t8.242400\t-0.881404\t-1.297273\t56.336010\t0.434000\t0.112000\n\t\n15:09:23.8\tlog_raw\tgps_raw\t#INSPVAXA,USB3,0,46.0,FINESTEERING,2107,281381.850,02000000,471d,15824;INS_ALIGNMENT_COMPLETE,INS_RTKFIXED,37.37091780548,126.72159081675,8.2350,22.3000,0.3759,0.2927,0.0016,-0.963689803,-1.123540768,33.630773348,0.4181,0.3018,0.5653,0.1129,0.0953,0.0850,0.2661,0.2404,5.1482,0f000001,0*05f2b425\n\tsystem status\tnormal 2 28.200000 0 0\trobot status\t66.939701\t87.412198\t8.235000\t-0.963690\t-1.123541\t56.369227\t0.427000\t0.104000\n\t\n15:09:24.3\tlog_raw\tgps_raw\t\tsystem status\tnormal 2 28.200000 0 0\trobot status\t67.066913\t87.582958\t8.229200\t-0.825346\t-0.852925\t56.373582\t0.453000\t0.083000\n\t\n15:09:24.8\tlog_raw\tgps_raw\t#DUALANTENNAHEADINGA,USB3,0,49.5,FINESTEERING,2107,281382.800,02000000,d426,15824;SOL_COMPUTED,NARROW_FLOAT,-1.000000000,34.756454468,-17.411163330,0.0,292.158599854,180.000000000,\"631T\",19,9,9,8,04,00,20,03*833ed280\n\tsystem status\tnormal 2 28.200000 0 0\trobot status\t67.206598\t87.772045\t8.224100\t-0.811726\t-0.925179\t56.378023\t0.567000\t-0.110000\n\t\n15:09:25.3\tlog_raw\tgps_raw\t#DUALANTENNAHEADINGA,USB3,0,48.0,FINESTEERING,2107,281383.300,02000000,d426,15824;SOL_COMPUTED,NARROW_FLOAT,-1.000000000,29.882240295,-12.166564941,0.0,299.295318604,180.000000000,\"631T\",20,9,9,8,04,00,20,03*2118f19e\n\tsystem status\tnormal 2 28.200000 0 0\trobot status\t67.350144\t87.966555\t8.219200\t-0.803825\t-1.261048\t56.294430\t0.574000\t-0.143000\n\t\n15:09:25.8\tlog_raw\tgps_raw\t#INSPVAXA,USB3,0,48.0,FINESTEERING,2107,281383.850,02000000,471d,15824;INS_ALIGNMENT_COMPLETE,INS_RTKFIXED,37.37092469082,126.72159717751,8.2117,22.3000,0.3710,0.2982,-0.0132,-1.063340683,-1.217564676,33.617373330,0.4191,0.3013,0.5725,0.1134,0.0950,0.0851,0.2661,0.2404,5.1497,0f000001,0*b9a6888a\n\tsystem status\tnormal 2 28.200000 0 0\trobot status\t67.503127\t88.176360\t8.211700\t-1.063341\t-1.217565\t56.382627\t0.590000\t-0.144000\n\t\n15:09:26.3\tlog_raw\tgps_raw\t\tsystem status\tnormal 2 28.200000 0 0\trobot status\t67.629071\t88.345427\t8.208400\t-0.916265\t-0.899647\t56.411155\t0.429000\t0.090000\n\t\n15:09:26.8\tlog_raw\tgps_raw\t\tsystem status\tnormal 2 28.200000 0 0\trobot status\t67.769097\t88.533025\t8.204900\t-0.678615\t-0.801791\t56.589829\t0.566000\t
